vi "吸光值辅助计算.vi"() -> (2 "X":dbl format="%#.6f", 3 "吸光值导出":u16(ring) items=["不导入", "标样一", "标样二", "标样三", "零点", "跨度"])   [LabVIEW 2016, in "斯坦道总磷.lvlib"]
panel:
  in  "确认":bool
  in  "导入至":u16(ring) items=["不导入", "标样一", "标样二", "标样三", "零点", "跨度"]
  in  "F1":dbl
  in  "F0":dbl
  in  "吸光值算法":enum16{"对数", "减法"}(ring)
  # "吸光值辅助计算"
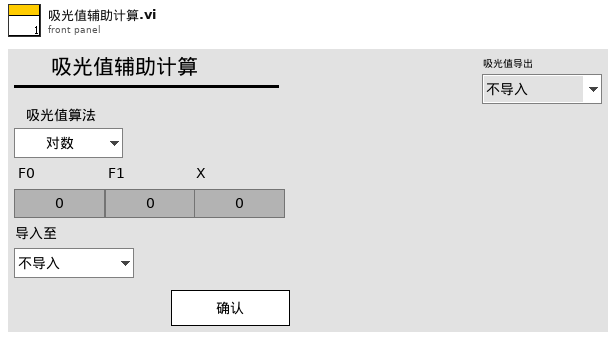
[diagram p1: front panel]
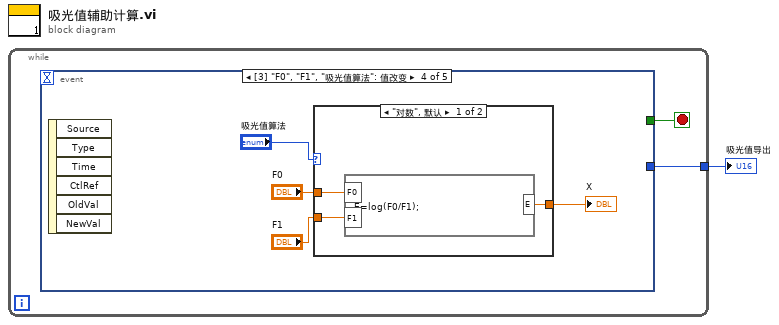
[diagram p0: block diagram]
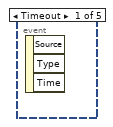
[diagram p2: hidden frame]
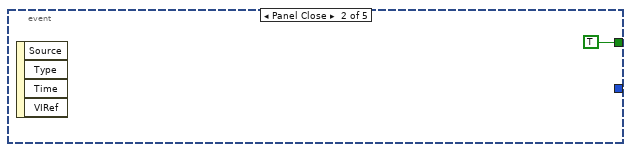
[diagram p3: hidden frame]
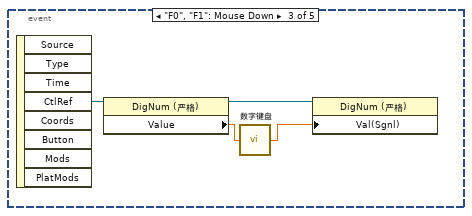
[diagram p4: hidden frame]
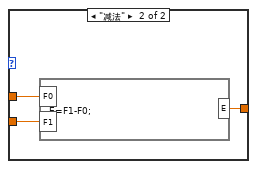
[diagram p5: hidden frame]
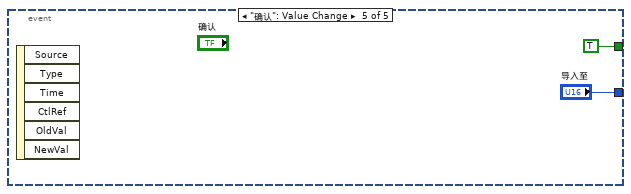
[diagram p6: hidden frame]
diagram:
  n1 = while {
    tunnel: [w2] -> w1
    stop <- w3 stop-if-true
    n2 = event shown="[3] \"F0\", \"F1\", \"吸光值算法\": 值改变" {
      selector: _ -> [_ _ _ _ _]
      dyn-events: _ -> [_ _ _ _ _]
      timeout: _ -> [_ _ _ _ _]
      tunnel: [_ TRUE _ _ TRUE] -> w3
      tunnel: [_ _ _ _ "导入至"] -> w2
      event Timeout {
        n3 = event-data() -> ()  [unwired: 1 in, 3 out]
      }
      event Panel Close {
        n4 = event-data() -> ()  [unwired: 1 in, 4 out]
      }
      event "F0", "F1": Mouse Down {
        n5 = event-data() -> ("CtlRef"=w8:refnum<vi>)  [unwired: 1 in, 7 out]
        n6 = property class="DigNum (严格)"(reference=w8) -> (reference out=w5:refnum<vi>, "Value"=w7:dbl)  [unwired: 1 in, 1 out]
        n7 = call "数字键盘.vi"("OldNumber"=w7) -> ("NewNumber"=w6:dbl)
        n8 = property class="DigNum (严格)"(reference=w5, "Val(Sgnl)"=w6) -> ()  [unwired: 1 in, 2 out]
      }
      event "F0", "F1", "吸光值算法": Value Change {
        n9 = event-data() -> ()  [unwired: 1 in, 6 out]
        n10 = case shown="\"对数\", 默认" "吸光值算法" {
          tunnel: "F0" -> [w15 w18]
          tunnel: "F1" -> [w14 w17]
          tunnel: [w13 w16] -> w12
          frame "对数", Default {
            n11 = formula code="E=log(F0/F1);"("F0"=w15, "F1"=w14) -> ("E"=w13:dbl)
          }
          frame "减法" {
            n12 = formula code="E=F1-F0;"("F0"=w18, "F1"=w17) -> ("E"=w16:dbl)
          }
        }
        "X" <- w12
      }
      event "确认": Value Change {
        n13 = event-data() -> ()  [unwired: 1 in, 6 out]
      }
    }
  }
  "吸光值导出" <- w1
